vi "Autonomous Independent.vi"   [LabVIEW 2016]
doc: "This VI is called when autonomous begins, and will automatically be terminated when autonomous ends. You can carry out timed or sensor driven robot movement independently without needing to return to the caller."
uses:
  <vilib>/Rock Robotics/WPI/SafetyOutput/WPI_SafetyOutputConfigMenu.ctl
  <vilib>/Rock Robotics/WPI/Utilities/WPI_GetSetVariantRefNum.vi
  <vilib>/Rock Robotics/Network Tables/NT Read String.vi
  <vilib>/Rock Robotics/WPI/Ultrasonic/WPI_SonarMB1010AnalogRefNum Registry Get.vi
  <vilib>/Rock Robotics/Network Tables/NT Read Number.vi
  <vilib>/Rock Robotics/WPI/Ultrasonic/WPI_SonarMB1010AnalogGetRange.vi
  <vilib>/Rock Robotics/WPI/RobotDrive/WPI_RobotDriveArcadeDrive_Standard(NoSaturation).vi
  <vilib>/Rock Robotics/Network Tables/NT Write Numeric Array.vi
types:
  T1 = typedef "WPI_JoystickDevRef.ctl" = cluster{"Device":T2}
  T2 = typedef "WPI_JoystickDeviceEnum.ctl" = enum16{"USB 0", "USB 1", "USB 2", "USB 3", "USB 4", "USB 5"}
  T3 = typedef "WPI_SafetyOutputConfigMenu.ctl" = enum16{"Enable", "Disable"}
  T4 = typedef "WPI_SonarMB1010AnalogDeviceRef.ctl" = cluster{"AIDeviceRef":T5, "Scaling factor (V/in)":dbl, "Average Bits":u8}
  T5 = typedef "WPI_AnalogChannelDevRef.ctl" = cluster{"DevStatus":errorcluster, "Analog Channel":T6}
  T6 = typedef "FPGA_AIChannel.ctl" = enum8{"AI 0", "AI 1", "AI 2", "AI 3", "AI MXP 0", "AI MXP 1", "AI MXP 2", "AI MXP 3", "Invalid"}
  T7 = typedef "WPI_RobotDriveDevRef.ctl" = cluster{"DevStatus":errorcluster, "Motors[]":T8[], "Square Inputs":bool, "Max Output":dbl}
  T8 = typedef "WPI_MotorControlDeviceRef.ctl" = cluster{"DeviceStatus":errorcluster, "Type":T9, "PWM":cluster{"PWM Channel":T10, "DeadBand":T11}, "CAN":cluster{"Device Number":u8, "SetOutput VI Ref":variant, "GetOutput VI Ref":variant, "Enable VI Ref":variant, "Disable VI Ref":variant, "Data":variant}, "Invert":bool}
  T9 = typedef "WPI_MotorControlType.ctl" = enum16{"PWM", "CAN"}
  T10 = typedef "FPGA_DIOPWMChannel.ctl" = enum8{"PWM 0", "PWM 1", "PWM 2", "PWM 3", "PWM 4", "PWM 5", "PWM 6", "PWM 7", "PWM 8", "PWM 9", "PWM MXP 0", "PWM MXP 1", "PWM MXP 2", "PWM MXP 3", "PWM MXP 4", "PWM MXP 5", "PWM MXP 6", "PWM MXP 7", "PWM MXP 8", "PWM MXP 9", "Invalid"}
  T11 = typedef "WPI_PWMDeadband.ctl" = cluster{"Name":string, "maxPositivePwm":i32, "minPositivePwm":i32, "centerPwm":i32, "maxNegativePwm":i32, "minNegativePwm":i32, "angularRange":u16}
  T12 = typedef "WPI_GyroDevRef.ctl" = cluster{"DevStatus":errorcluster, "Analog Channel":T6, "Offset":dbl, "Gain (VoltsPerDegree/Second)":dbl, "Gyro Type":enum16{"Analog", "XRS450"}, "Handle":i32, "SPI Bus":T13, "Device Found":bool, "Sample Rate":dbl, "Calibrate On Open":bool}
  T13 = typedef "spi_bus.ctl" = enum16{"SPI On-Board, CS0", "SPI On-Board, CS1", "SPI On-Board, CS2", "SPI On-Board, CS3", "SPI MXP", "Invalid"}
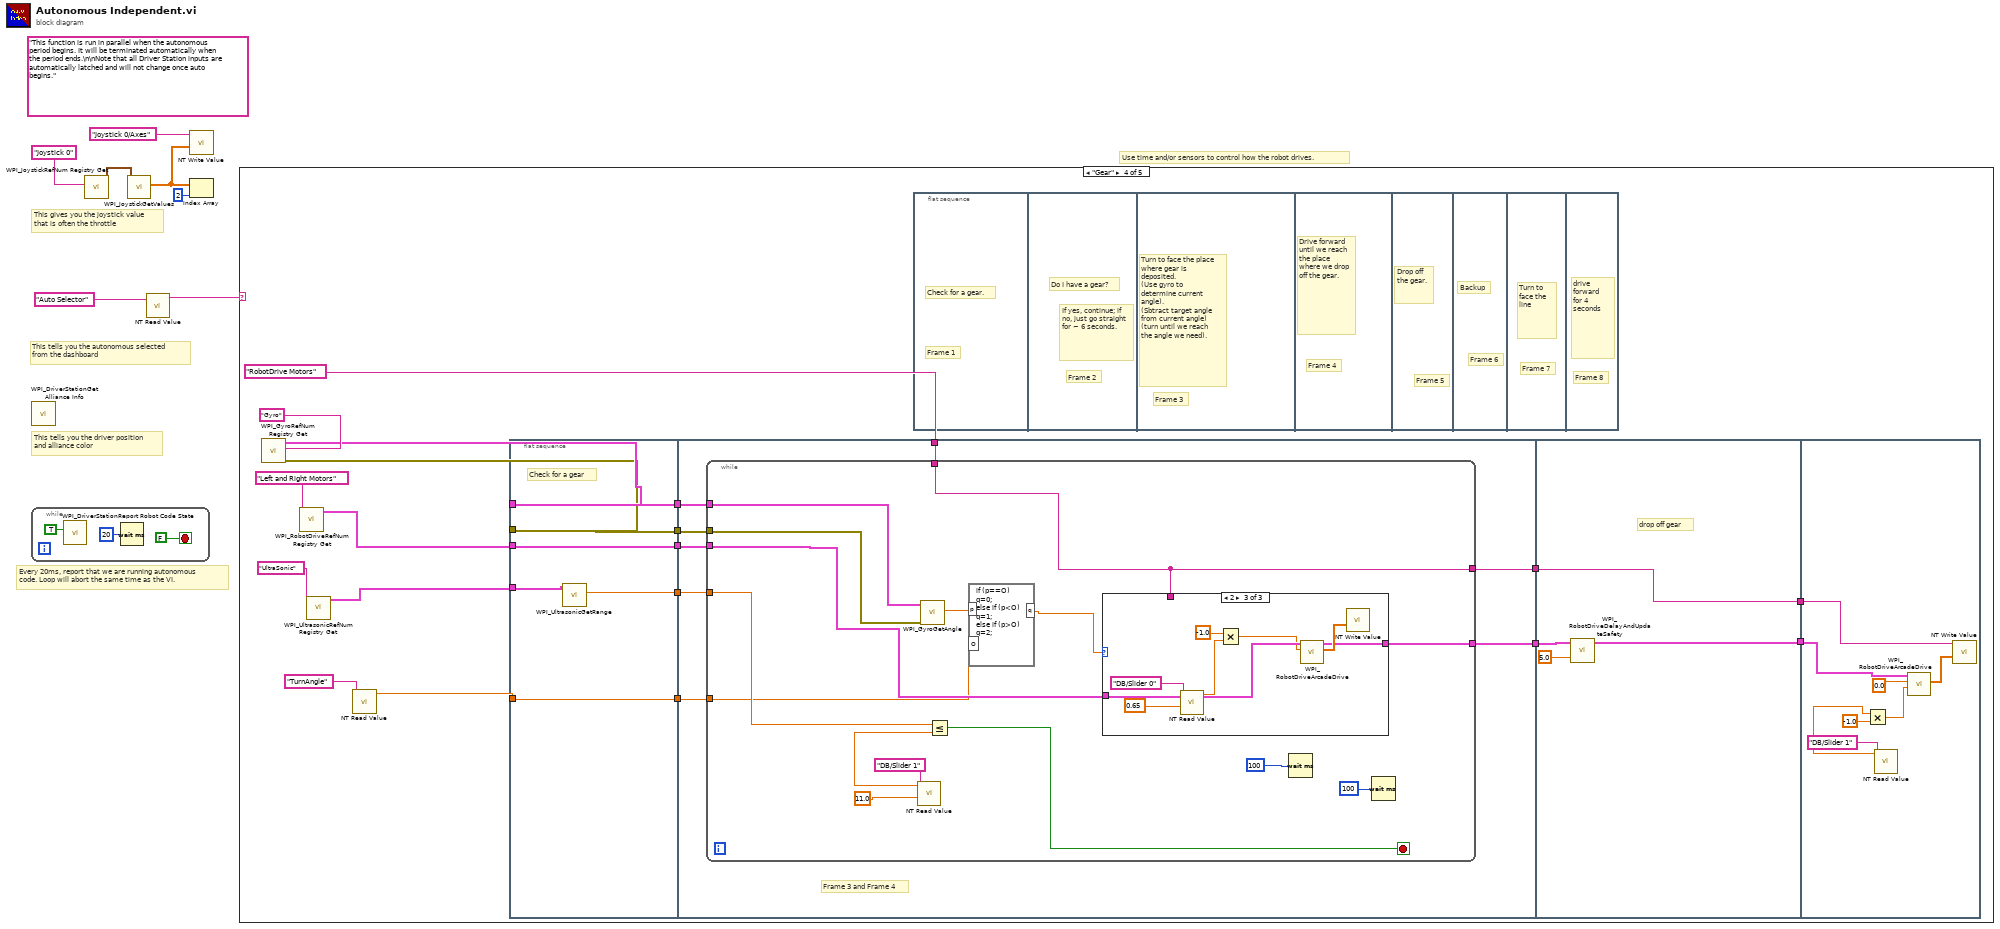
[diagram p0: block diagram]
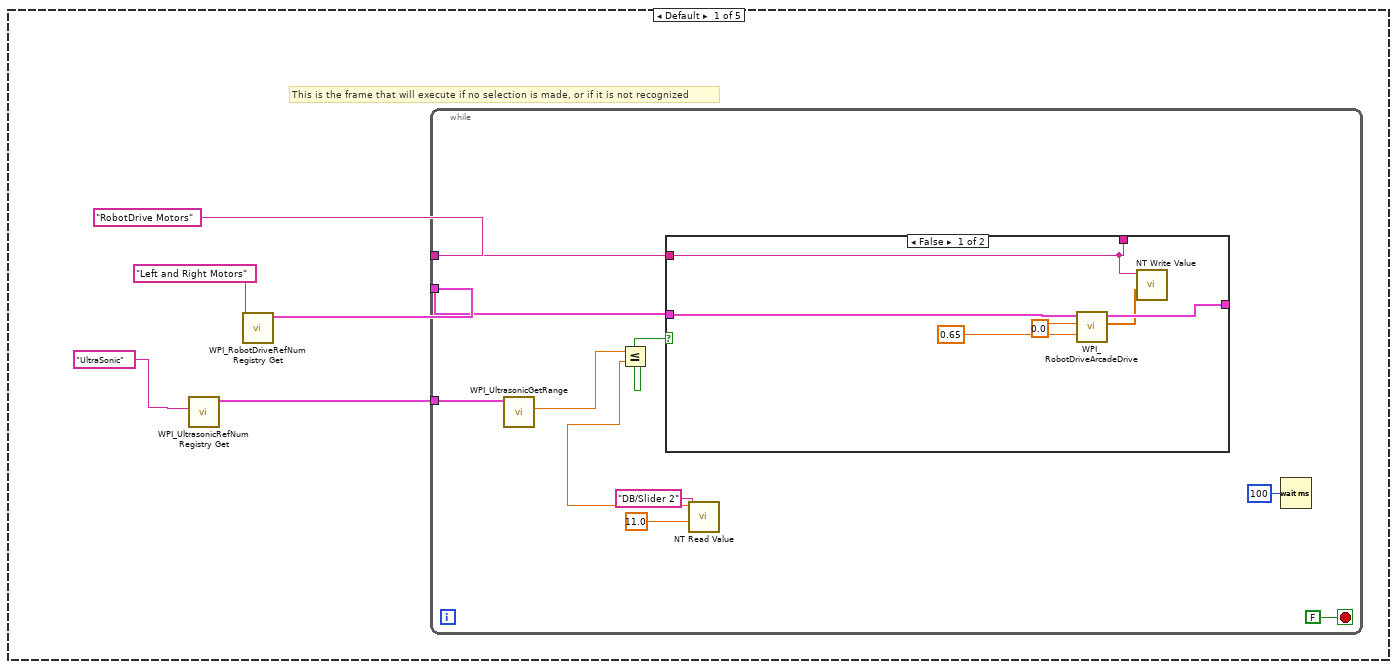
[diagram p2: hidden frame]
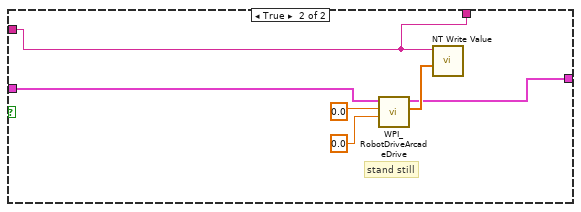
[diagram p3: hidden frame]
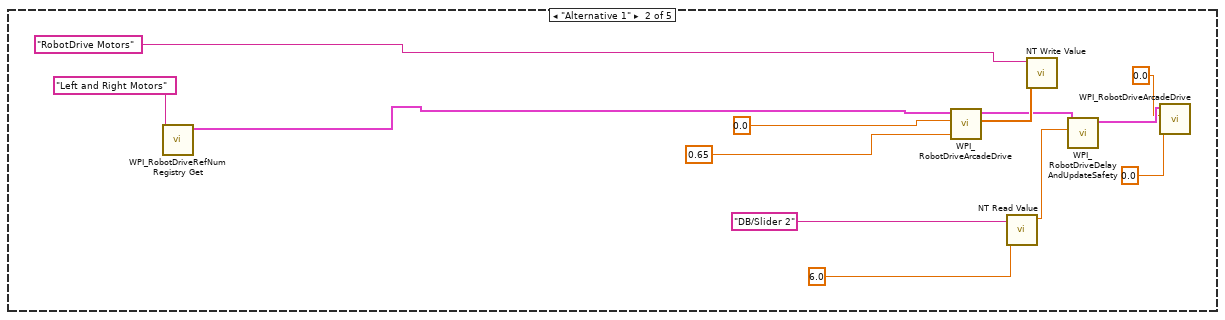
[diagram p4: hidden frame]
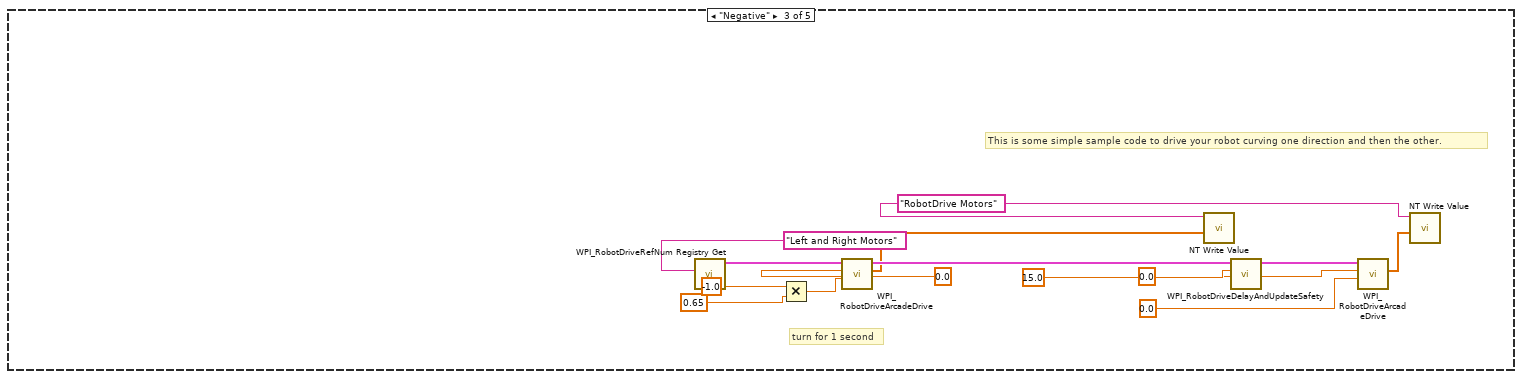
[diagram p5: hidden frame]
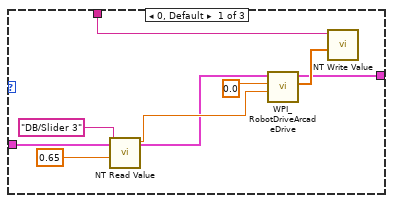
[diagram p6: hidden frame]
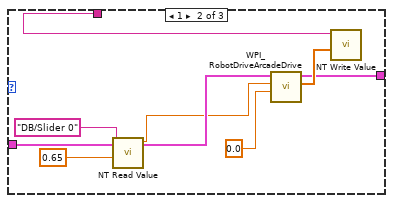
[diagram p7: hidden frame]
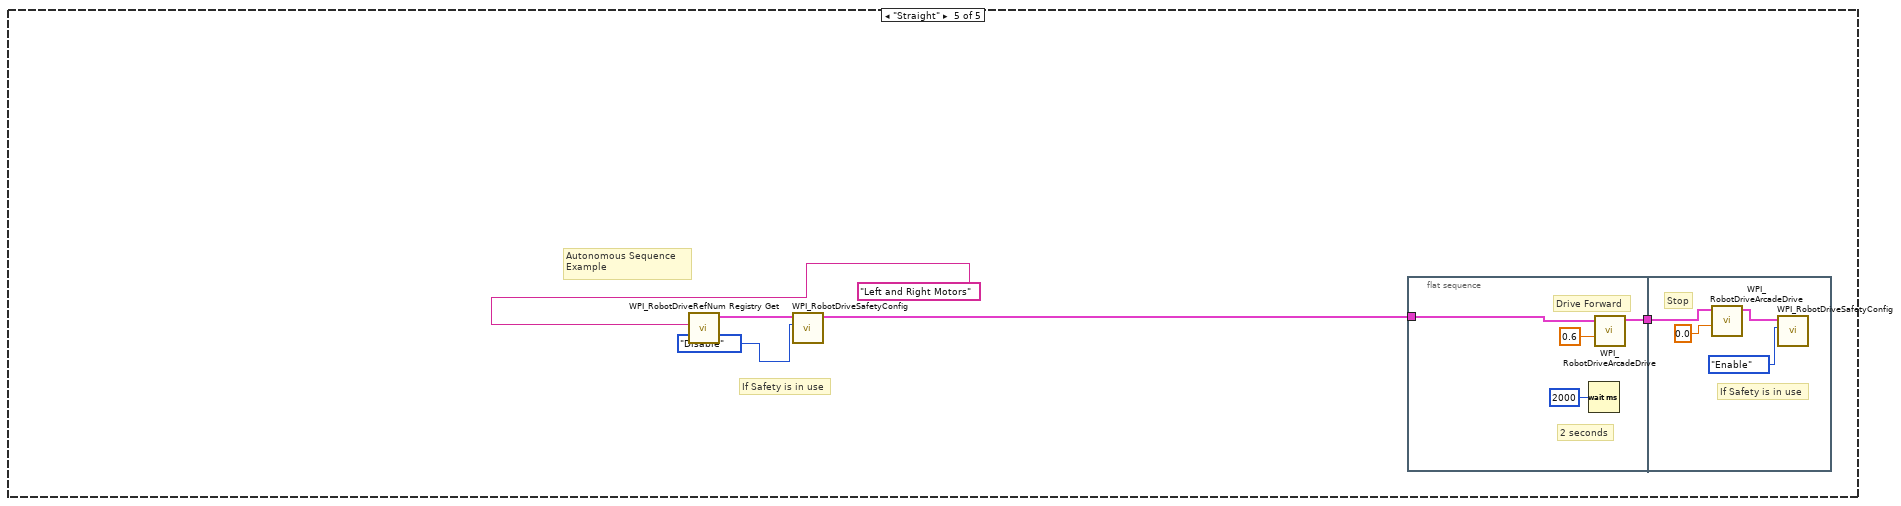
[diagram p8: hidden frame]
diagram:
  (unwired) "This function is run in parallel when the autonomous period begins. It will be terminated automatically when the period ends.\n\nNote that all Driver Station inputs are automatically latched and will not change once auto begins."
  # "This tells you the autonomous selected\nfrom the dashboard"
  # "Every 20ms, report that we are running autonomous\ncode. Loop will abort the same time as the VI."
  # "This gives you the joystick value\nthat is often the throttle"
  # "Use time and/or sensors to control how the robot drives."
  # "This tells you the driver position\nand alliance color"
  n1 = while {
    stop <- FALSE stop-if-true
    n2 = call <vilib>:"WPI_DriverStationReport Robot Code State.vi"("Autonomous"=TRUE) -> ()  [unwired: 10 in, 1 out]
    n3 = Wait (ms)(milliseconds to wait=u32 20) -> ()  [unwired: 1 out]
  }
  n4 = call <vilib>:"WPI_DriverStationGet Alliance Info.vi"() -> ()  [unwired: 12 out]
  n5 = call <vilib>:"WPI_JoystickRefNum Registry Get.vi"("refnum name"="Joystick 0") -> ("JoystickDevRef"=w6:T1)  [unwired: 1 in, 9 out]
  n6 = call <vilib>:"WPI_JoystickGetValues.vi"("JoystickDevRef"=w6) -> ("Axes"=w2:dbl[])  [unwired: 6 in, 4 out]
  n7 = call-poly <vilib>:"NT Read Value.vi"("Name"="Auto Selector") -> ("String"=w3:string)  [unwired: 9 in, 1 out]
  n8 = call-poly <vilib>:"NT Write Value.vi"("Numeric Array"=w2, "Name"="Joystick 0/Axes") -> ()  [unwired: 9 in, 1 out]
  n9 = Index Array(array=w2, index=2) -> ()  [unwired: 1 out]
  n10 = case shown="\"Gear\"" w3 {
    frame Default {
      # "This is the frame that will execute if no selection is made, or if it is not recognized"
      n11 = call-poly <vilib>:"WPI_UltrasonicRefNum Registry Get.vi"("refnum name"="UltraSonic") -> ("SonarMB1010AnalogDevRef"=w11:T4)  [unwired: 9 in, 1 out]
      n12 = call <vilib>:"WPI_RobotDriveRefNum Registry Get.vi"("refnum name"="Left and Right Motors") -> ("RobotDriveDevRef"=w12:T7)  [unwired: 1 in, 9 out]
      n13 = while {
        tunnel: "RobotDrive Motors" ("Name") -> [w24]
        tunnel: w12 -> [w23]
        tunnel: w11 -> [w21]
        stop <- FALSE stop-if-true
        n14 = call-poly <vilib>:"WPI_UltrasonicGetRange.vi"("SonarMB1010AnalogDevRef"=w21) -> ("Distance"=w22:dbl)  [unwired: 8 in, 2 out]
        n15 = call-poly <vilib>:"NT Read Value.vi"("Default Value"=11.0, "Name"="DB/Slider 2") -> ("Numeric"=w16:dbl)  [unwired: 8 in, 1 out]
        n16 = Less Or Equal?(x=w22, y=w16) -> (x <= y?=w25:bool)
        n17 = case shown="False" w25 {
          tunnel: w24 -> [w30 w32]
          tunnel: [w30 w32] -> _
          tunnel: w23 -> [w29 w34]
          tunnel: [w28 w33] -> _
          frame False {
            n18 = call-poly <vilib>:"WPI_RobotDriveArcadeDrive.vi"("Y axis value"=0.65, "X axis value"=0.0, "RobotDriveDevRef"=w29) -> ("Motor Values"=w26:dbl[], "RobotDriveDevRef"=w28:T7)  [unwired: 1 in, 6 out]
            n19 = call-poly <vilib>:"NT Write Value.vi"("Numeric Array"=w26, "Name"=w30) -> ()  [unwired: 9 in, 1 out]
          }
          frame True {
            # "stand still"
            n20 = call-poly <vilib>:"WPI_RobotDriveArcadeDrive.vi"("Y axis value"=0.0 ("X axis value"), "X axis value"=0.0, "RobotDriveDevRef"=w34) -> ("Motor Values"=w37:dbl[], "RobotDriveDevRef"=w33:T7)  [unwired: 1 in, 6 out]
            n21 = call-poly <vilib>:"NT Write Value.vi"("Numeric Array"=w37, "Name"=w32) -> ()  [unwired: 9 in, 1 out]
          }
        }
        n22 = Wait (ms)(milliseconds to wait=u32 100) -> ()  [unwired: 1 out]
      }
    }
    frame "Alternative 1" {
      n23 = call <vilib>:"WPI_RobotDriveRefNum Registry Get.vi"("refnum name"="Left and Right Motors") -> ("RobotDriveDevRef"=w46:T7)  [unwired: 1 in, 9 out]
      n24 = call-poly <vilib>:"WPI_RobotDriveArcadeDrive.vi"("Y axis value"=0.65, "X axis value"=0.0, "RobotDriveDevRef"=w46) -> ("Motor Values"=w47:dbl[], "RobotDriveDevRef"=w44:T7)  [unwired: 1 in, 6 out]
      n25 = call-poly <vilib>:"NT Read Value.vi"("Default Value"=6.0, "Name"="DB/Slider 2") -> ("Numeric"=w40:dbl)  [unwired: 8 in, 1 out]
      n26 = call-poly <vilib>:"NT Write Value.vi"("Numeric Array"=w47, "Name"="RobotDrive Motors") -> ()  [unwired: 9 in, 1 out]
      n27 = call <vilib>:"WPI_RobotDriveDelayAndUpdateSafety.vi"("Delay (s)"=w40, "RobotDriveDevRef"=w44) -> ("RobotDriveDevRef 2"=w43:T7)  [unwired: 8 in, 1 out]
      n28 = call-poly <vilib>:"WPI_RobotDriveArcadeDrive.vi"("Y axis value"=0.0, "X axis value"=0.0, "RobotDriveDevRef"=w43) -> ()  [unwired: 1 in, 8 out]
    }
    frame "Negative" {
      w55 = "RobotDrive Motors" ("Name")
      # "This is some simple sample code to drive your robot curving one direction and then the other."
      # "turn for 1 second"
      n29 = call <vilib>:"WPI_RobotDriveRefNum Registry Get.vi"("refnum name"="Left and Right Motors") -> ("RobotDriveDevRef"=w64:T7)  [unwired: 1 in, 9 out]
      n30 = Multiply(x=-1.0, y=0.65 ("Default Value")) -> (x*y=w52:dbl)
      n31 = call-poly <vilib>:"WPI_RobotDriveArcadeDrive.vi"("Y axis value"=w52, "X axis value"=0.0, "RobotDriveDevRef"=w64) -> ("Motor Values"=w54:dbl[], "RobotDriveDevRef"=w60:T7)  [unwired: 1 in, 6 out]
      n32 = call-poly <vilib>:"NT Write Value.vi"("Numeric Array"=w54, "Name"=w55) -> ()  [unwired: 9 in, 1 out]
      n33 = call <vilib>:"WPI_RobotDriveDelayAndUpdateSafety.vi"("Delay (s)"=15.0, "RobotDriveDevRef"=w60) -> ("RobotDriveDevRef 2"=w61:T7)  [unwired: 8 in, 1 out]
      n34 = call-poly <vilib>:"WPI_RobotDriveArcadeDrive.vi"("Y axis value"=0.0 ("X axis value"), "X axis value"=0.0, "RobotDriveDevRef"=w61) -> ("Motor Values"=w56:dbl[])  [unwired: 1 in, 7 out]
      n35 = call-poly <vilib>:"NT Write Value.vi"("Numeric Array"=w56, "Name"=w55) -> ()  [unwired: 9 in, 1 out]
    }
    frame "Gear" {
      n36 = call <vilib>:"WPI_GyroRefNum Registry Get.vi"("refnum name"="Gyro") -> ("error out"=w68:errorcluster, "GyroDevRef"=w74:T12)  [unwired: 9 in]
      n37 = call <vilib>:"WPI_RobotDriveRefNum Registry Get.vi"("refnum name"="Left and Right Motors") -> ("RobotDriveDevRef"=w72:T7)  [unwired: 1 in, 9 out]
      n38 = call-poly <vilib>:"WPI_UltrasonicRefNum Registry Get.vi"("refnum name"="UltraSonic") -> ("SonarMB1010AnalogDevRef"=w69:T4)  [unwired: 9 in, 1 out]
      n39 = call-poly <vilib>:"NT Read Value.vi"("Name"="TurnAngle") -> ("Numeric"=w65:dbl)  [unwired: 9 in, 1 out]
      n40 = flat-sequence {
        tunnel: w74 -> [w89]
        tunnel: [w89] -> w83
        tunnel: [w88] -> w82
        tunnel: w72 -> [w88]
        tunnel: w69 -> [w87]
        tunnel: [w86] -> w81
        tunnel: w68 -> [w86]
        tunnel: [w85] -> w80
        tunnel: [w84] -> w67
        tunnel: w65 -> [w84]
        tunnel: w83 -> [w97]
        tunnel: w82 -> [w96]
        tunnel: "RobotDrive Motors" ("Name") -> [w95]
        tunnel: w81 -> [w94]
        tunnel: w80 -> [w93]
        tunnel: [w92] -> w79
        tunnel: [w91] -> w78
        tunnel: w67 -> [w90]
        tunnel: w79 -> [w140]
        tunnel: w78 -> [w139]
        tunnel: [w139] -> w77
        tunnel: [w138] -> w76
        tunnel: w77 -> [w145]
        tunnel: w76 -> [w144]
        frame #0 {
          # "Check for a gear"
          n41 = call-poly <vilib>:"WPI_UltrasonicGetRange.vi"("SonarMB1010AnalogDevRef"=w87) -> ("Distance"=w85:dbl)  [unwired: 8 in, 2 out]
        }
        frame #1 {
          # "Frame 3 and Frame 4"
          n42 = while {
            tunnel: w97 -> [w111]
            tunnel: w96 -> [w110]
            tunnel: w95 -> [w100]
            tunnel: w94 -> [w109]
            tunnel: w93 -> [w103]
            tunnel: [w101] -> w92
            tunnel: [w100] -> w91
            tunnel: w90 -> [w99]
            stop <- w102 stop-if-true
            n43 = call-poly <vilib>:"NT Read Value.vi"("Default Value"=11.0 ("y"), "Name"="DB/Slider 1") -> ("Numeric"=w104:dbl)  [unwired: 8 in, 1 out]
            n44 = call <vilib>:"WPI_GyroGetAngle.vi"("error in"=w109, "GyroDevRef"=w111) -> ("Angle"=w108:dbl)  [unwired: 5 in, 4 out]
            n45 = Less Or Equal?(x=w103, y=w104) -> (x <= y?=w102:bool)
            n46 = formula code="if (p==O)\nq=0;\nelse if (p<O)\nq=1;\nelse if (p>O)\nq=2;"("p"=w108, "O"=w99) -> ("q"=w107:dbl)
            n47 = case shown="2" w107 {
              tunnel: w110 -> [w115 w125 w133]
              tunnel: w100 -> [w114 w124 _]
              tunnel: [w113 w121 w129] -> w101
              frame 0, Default {
                n48 = call-poly <vilib>:"NT Read Value.vi"("Default Value"=0.65, "Name"="DB/Slider 3") -> ("Numeric"=w118:dbl)  [unwired: 8 in, 1 out]
                n49 = call-poly <vilib>:"WPI_RobotDriveArcadeDrive.vi"("Y axis value"=w118, "X axis value"=0.0, "RobotDriveDevRef"=w115) -> ("Motor Values"=w117:dbl[], "RobotDriveDevRef"=w113:T7)  [unwired: 1 in, 6 out]
                n50 = call-poly <vilib>:"NT Write Value.vi"("Numeric Array"=w117, "Name"=w114) -> ()  [unwired: 9 in, 1 out]
              }
              frame 1 {
                n51 = call-poly <vilib>:"NT Read Value.vi"("Default Value"=0.65, "Name"="DB/Slider 0") -> ("Numeric"=w123:dbl)  [unwired: 8 in, 1 out]
                n52 = call-poly <vilib>:"WPI_RobotDriveArcadeDrive.vi"("Y axis value"=0.0, "X axis value"=w123, "RobotDriveDevRef"=w125) -> ("Motor Values"=w126:dbl[], "RobotDriveDevRef"=w121:T7)  [unwired: 1 in, 6 out]
                n53 = call-poly <vilib>:"NT Write Value.vi"("Numeric Array"=w126, "Name"=w124) -> ()  [unwired: 9 in, 1 out]
              }
              frame 2 {
                n54 = call-poly <vilib>:"NT Read Value.vi"("Default Value"=0.65, "Name"="DB/Slider 0") -> ("Numeric"=w132:dbl)  [unwired: 8 in, 1 out]
                n55 = Multiply(x=-1.0, y=w132) -> (x*y=w131:dbl)
                n56 = call-poly <vilib>:"WPI_RobotDriveArcadeDrive.vi"("X axis value"=w131, "RobotDriveDevRef"=w133) -> ("Motor Values"=w136:dbl[], "RobotDriveDevRef"=w129:T7)  [unwired: 2 in, 6 out]
                n57 = call-poly <vilib>:"NT Write Value.vi"("Numeric Array"=w136) -> ()  [unwired: 10 in, 1 out]
              }
            }
            n58 = Wait (ms)(milliseconds to wait=u32 100) -> ()  [unwired: 1 out]
          }
          n59 = Wait (ms)(milliseconds to wait=u32 100) -> ()  [unwired: 1 out]
        }
        frame #2 {
          # "drop off gear"
          n60 = call <vilib>:"WPI_RobotDriveDelayAndUpdateSafety.vi"("Delay (s)"=5.0, "RobotDriveDevRef"=w140) -> ("RobotDriveDevRef 2"=w138:T7)  [unwired: 8 in, 1 out]
        }
        frame #3 {
          n61 = call-poly <vilib>:"NT Read Value.vi"("Name"="DB/Slider 1") -> ("Numeric"=w143:dbl)  [unwired: 9 in, 1 out]
          n62 = Multiply(x=w143, y=-1.0) -> (x*y=w141:dbl)
          n63 = call-poly <vilib>:"WPI_RobotDriveArcadeDrive.vi"("Y axis value"=w141, "X axis value"=0.0, "RobotDriveDevRef"=w144) -> ("Motor Values"=w147:dbl[])  [unwired: 1 in, 7 out]
          n64 = call-poly <vilib>:"NT Write Value.vi"("Numeric Array"=w147, "Name"=w145) -> ()  [unwired: 9 in, 1 out]
        }
      }
      n65 = flat-sequence {
        frame #0 {
          # "Frame 1"
          # "Check for a gear."
        }
        frame #1 {
          # "Frame 2"
          # "If yes, continue; if no, just go straight for ~ 6 seconds."
          # "Do I have a gear?"
        }
        frame #2 {
          # "Frame 3"
          # "Turn to face the place where gear is deposited.\n(Use gyro to determine current angle).\n(Sbtract target angle from current angle)\n(turn until we reach the angle we need)."
        }
        frame #3 {
          # "Drive forward until we reach the place where we drop off the gear."
          # "Frame 4"
        }
        frame #4 {
          # "Frame 5"
          # "Drop off the gear."
        }
        frame #5 {
          # "Frame 6"
          # "Backup"
        }
        frame #6 {
          # "Frame 7"
          # "Turn to face the line"
        }
        frame #7 {
          # "Frame 8"
          # "drive forward for 4 seconds"
        }
      }
    }
    frame "Straight" {
      # "If Safety is in use"
      # "Autonomous Sequence\nExample"
      n66 = call <vilib>:"WPI_RobotDriveRefNum Registry Get.vi"("refnum name"="Left and Right Motors") -> ("RobotDriveDevRef"=w151:T7)  [unwired: 9 in, 1 out]
      n67 = call <vilib>:"WPI_RobotDriveSafetyConfig.vi"("mode"=WPI_SafetyOutputConfigMenu."Disable", "RobotDriveDevRef"=w151) -> ("RobotDriveDevRef"=w150:T7)  [unwired: 8 in, 1 out]
      n68 = flat-sequence {
        tunnel: w150 -> [w155]
        tunnel: [w154] -> w153
        tunnel: w153 -> [w158]
        frame #0 {
          # "2 seconds"
          # "Drive Forward"
          n69 = Wait (ms)(milliseconds to wait=u32 2000) -> ()  [unwired: 1 out]
          n70 = call-poly <vilib>:"WPI_RobotDriveArcadeDrive.vi"("Y axis value"=0.6 ("Left axis value"), "RobotDriveDevRef"=w155) -> ("RobotDriveDevRef"=w154:T7)  [unwired: 7 in, 2 out]
        }
        frame #1 {
          # "If Safety is in use"
          # "Stop"
          n71 = call-poly <vilib>:"WPI_RobotDriveArcadeDrive.vi"("Y axis value"=0.0 ("Left axis value"), "RobotDriveDevRef"=w158) -> ("RobotDriveDevRef"=w159:T7)  [unwired: 7 in, 2 out]
          n72 = call <vilib>:"WPI_RobotDriveSafetyConfig.vi"("mode"=WPI_SafetyOutputConfigMenu."Enable", "RobotDriveDevRef"=w159) -> ()  [unwired: 8 in, 2 out]
        }
      }
    }
  }
